vi "Result to DBL.vi"(8 "error in (no error)":errorcluster, 11 "Mag Lab Result":refnum<class "Mag Lab Result.lvclass">) -> (0 "error out":errorcluster, 2 "Value":dbl, 3 "Mag Lab Result out":refnum<class "Mag Lab Result.lvclass">)   [LabVIEW 2015]
uses:
  Mag Lab Result.lvclass
  DBL Result/DBL Result.lvclass
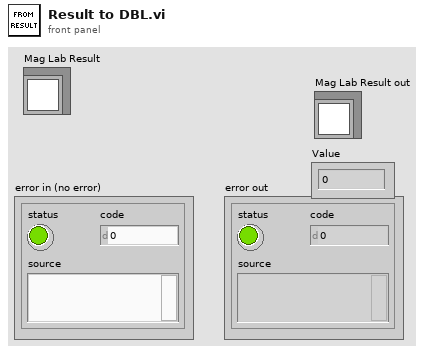
[diagram p1: front panel]
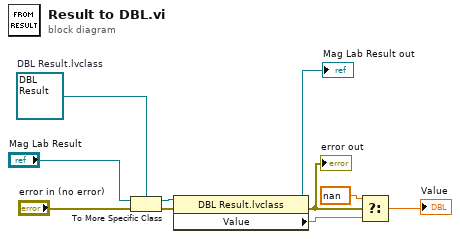
[diagram p0: block diagram]
diagram:
  w10 = refnum<class "DBL Result.lvclass"> refnum  # DBL Result.lvclass
  n1 = To More Specific Class(target class=w10, reference="Mag Lab Result", error in="error in (no error)") -> (specific class reference=w5:refnum<class "DBL Result.lvclass">, error out=w7:errorcluster)
  n2 = property class="DBL Result.lvclass"(reference=w5, error in=w7) -> (reference out=→"Mag Lab Result out":refnum<class "DBL Result.lvclass">, error out=w2:errorcluster, "Value"=w4:dbl)
  "error out" <- w2
  n3 = Select(t=nan, s=w2, f=w4) -> (s? t:f=→"Value":dbl)
